vi "DHE_Lib_get_elapsed.vi"(11 "error in (no error)":errorcluster) -> (6 "elapsed":i32, 8 "darktime":i32, 15 "error out":errorcluster)   [LabVIEW 2016]
doc: "This VI opens (Flag=1) or closes (Flag=0) the instrument shutter."
uses:
  c/lib/libgendhe.so
panel:
  in  "dtime":i32
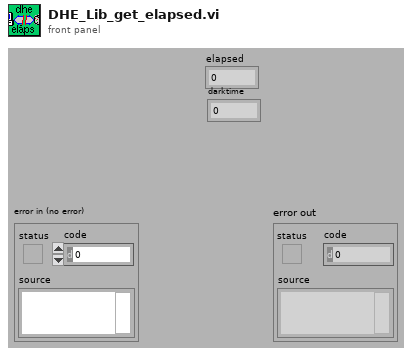
[diagram p1: front panel]
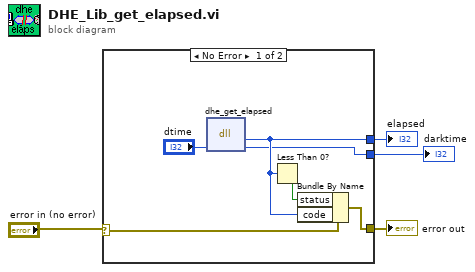
[diagram p0: block diagram]
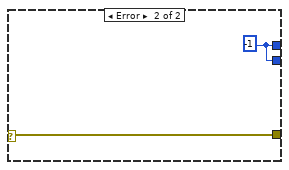
[diagram p2: hidden frame]
diagram:
  n1 = case shown="No Error" "error in (no error)" {
    selector: "error in (no error)" -> [w8 w12]
    tunnel: [w7 w12] -> w4
    tunnel: [w9 w11] -> w2
    tunnel: [w5 w11] -> w1
    frame No Error {
      n2 = dll-call lib="home/sispi/panview/PAN/Modules/DHE/private/c/lib/libgendhe.so" fn="dhe_get_elapsed"("darktime"="dtime") -> ("return type"=w9:i32, "darktime"=w5:i32)  [unwired: 3 in, 2 out]
      n3 = Less Than 0?(x=w9) -> (x < 0?=w10:bool)
      n4 = Bundle By Name(cluster=w8, "status"=w10, "code"=w9) -> (w7:errorcluster)
    }
    frame Error {
      w11 = -1
    }
  }
  "error out" <- w4
  "elapsed" <- w2
  "darktime" <- w1
